vi "ROSPublisher.vi"(2 "Response":T1, 3 "ROS":T2={"topic port"=1236, "Node"="/labview", "topic"="/robot/head/command_head_nod", "type"="std_msgs/Bool", "node port"=7000, "error "={"status"=FALSE, "code"=0, "source"=""}, "Direction"=enum."Publisher", "Update (ms)"=1, "FIFO size"=1}) -> ()   [LabVIEW 2012]
doc: "Opens new ports for publishers, updates publishers with master, and closes publishers"
uses:
  <userlib>/ROS for LabVIEW Software/ROS/Code/SubVIs/_ROSControl.ctl
  <userlib>/ROS for LabVIEW Software/ROS/Code/SubVIs/_ROSDirection.ctl
  <userlib>/ROS for LabVIEW Software/ROS/Code/_ROSDefinition.vi
panel:
  out "ports":i32[](array[numeric])
  out "Queue log":string
  out "Watchdog":i32
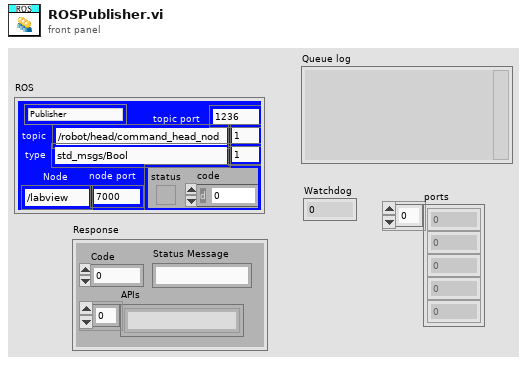
[diagram p1: front panel]
types:
  T1 = cluster{"Code":i32, "Status Message":string, "APIs":string[]}
  T2 = typedef "_ROSControl.ctl" = cluster{"topic port":u16, "Node":string, "topic":string, "type":string, "node port":u16, "error ":errorcluster, "Direction":T3, "Update (ms)":u16, "FIFO size":u16}
  T3 = typedef "_ROSDirection.ctl" = enum16{"Node", "Publisher", "Subscriber", "ServiceClient", "ServiceProvider"}
  T4 = enum16{"Reset Log", "Add Client", "Remove Client", "Add Task"}
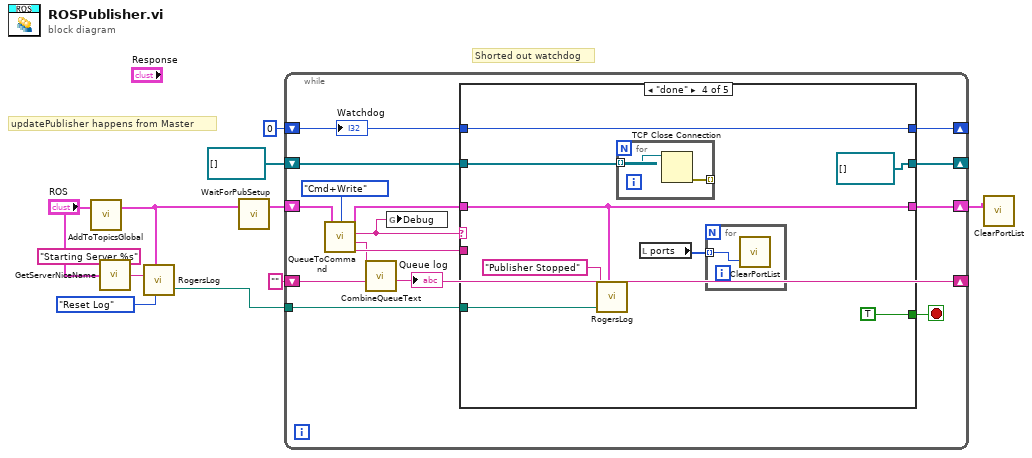
[diagram p0: block diagram]
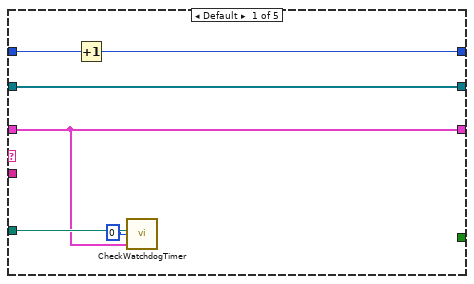
[diagram p2: hidden frame]
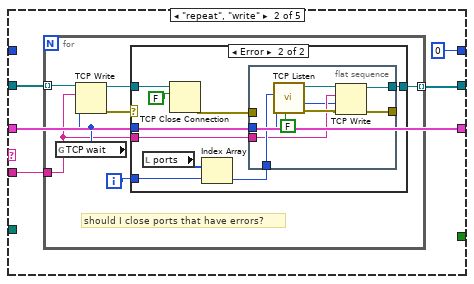
[diagram p3: hidden frame]
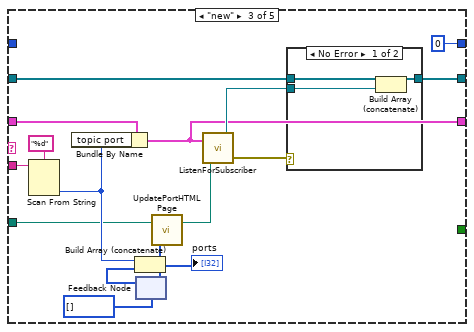
[diagram p5: hidden frame]
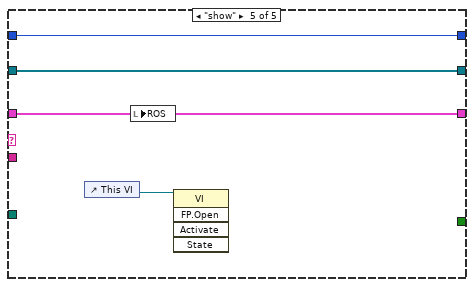
[diagram p7: hidden frame]
diagram:
  # "Shorted out watchdog"
  # "updatePublisher happens from Master"
  n1 = call <userlib>:"AddToTopicsGlobal.vi"("ROS in"="ROS") -> ("ROS out"=w1:T2)  [unwired: 2 in]
  n2 = call <userlib>:"GetServerNiceName.vi"("ROS"="ROS", "Text to add"="Starting Server %s") -> ("String"=w10:string)
  n3 = call <userlib>:"RogersLog.vi"("Text to add"=w10, "ROS"=w1, "Task"=T4."Reset Log") -> ("LogPath out"=w7:path)  [unwired: 2 in, 1 out]
  n4 = call <userlib>:"WaitForPubSetup.vi"("ROS in"=w1) -> ("ROS out"=w5:T2)  [unwired: 2 in]
  n5 = while {
    tunnel: w7 -> [w23]
    shift-right: [w21] -> _
    shift-left: 0 ("timeout ms (wait forever: -1)") -> [w22]
    shift-right: [w20] -> _
    shift-left: refnum<k5>[] [] -> [w26]
    shift-right: [w17] -> _
    shift-left: "" ("New List") -> [w19]
    shift-right: [w14] -> w2
    shift-left: w5 -> [w16]
    stop <- w24 stop-if-true
    n6 = call <userlib>:"QueueToCommand.vi"("ROS"=w16, "Check"=enum16{"Cmd+Write", "FIFO", "CMD", "CMD /wait"}."Cmd+Write") -> ("ROS out"=w15:T2, "Command"=w12:string, "Queue log"=w18:string, "data"=w25:string)  [unwired: 1 in]
    n7 = call <userlib>:"CombineQueueText.vi"("Old List"=w19, "Queue In"=w18) -> ("New List"=w17:string)  [unwired: 1 in]
    "Queue log" <- w17
    n8 = global write "_ROSDefinition.vi" "Debug"(w12) -> ()
    n9 = case shown="\"done\"" w12 {
      tunnel: w26 -> [w31 w36 w74 w84 w94]
      tunnel: w25 -> [_ w33 w76 _ _]
      tunnel: [_ _ _ TRUE _] -> w24
      tunnel: w23 -> [w29 _ w65 w88 _]
      tunnel: w22 -> [w32 _ _ w86 w95]
      tunnel: [w30 0 ("timeout ms (wait forever: -1)") 0 ("timeout ms (wait forever: -1)") w86 w95] -> w21
      tunnel: w15 -> [w27 w34 w67 w82 w93]
      tunnel: [w31 w35 w72 refnum<k5>[] [] w94] -> w20
      tunnel: [w27 w34 w63 w82 w93] -> w14
      frame Default {
        n10 = Increment(x=w32) -> (x+1=w30:i32)
        n11 = call <userlib>:"CheckWatchdogTimer.vi"("ROS"=w27, "itteration"=0, "LogPath in"=w29) -> ()  [unwired: 3 in]
      }
      frame "repeat", "write" {
        n12 = for {
          tunnel: w36 -> [w44] mode=indexing
          tunnel: w33 -> [w38]
          tunnel: [w41] -> w35 mode=indexing
          i -> [w40]
          # "should I close ports that have errors?"
          n13 = global read "_ROSDefinition.vi" "TCP wait"() -> (w39:i32)
          n14 = TCP Write(connection ID=w44, data in=w38, 9:w39) -> (connection ID out=w42:refnum<k5>, error out=w43:errorcluster)  [unwired: 1 in, 1 out]
          n15 = case shown="Error" w43 {
            tunnel: w42 -> [w45 w54]
            tunnel: [w45 w52] -> w41
            tunnel: w40 -> [_ w50]
            tunnel: w39 -> [_ w47]
            tunnel: w38 -> [_ w46]
            frame No Error {
            }
            frame Error {
              n16 = local read "ports"() -> (w51:i32[])
              n17 = TCP Close Connection(connection ID=w54, abort (F)=FALSE) -> (error out=w48:errorcluster)  [unwired: 1 in, 1 out]
              n18 = Index Array(array=w51, index=w50) -> (element=w49:i32)
              n19 = flat-sequence {
                tunnel: [w58] -> w52
                tunnel: w49 -> [w62]
                tunnel: w47 -> [w55]
                tunnel: w48 -> [_]
                tunnel: [w60] -> _
                tunnel: w46 -> [w57]
                frame #0 {
                  n20 = call <vilib>:"TCP Listen.vi"("resolve remote address (T)"=FALSE, "timeout ms (wait forever: -1)"=w55, "port"=w62) -> ("error out"=w61:errorcluster, "connection ID"=w59:refnum<k5>)  [unwired: 4 in, 3 out]
                  n21 = TCP Write(connection ID=w59, data in=w57, error in (no error)=w61, 9:w55) -> (connection ID out=w58:refnum<k5>, error out=w60:errorcluster)  [unwired: 1 out]
                }
              }
            }
          }
        }
      }
      frame "new" {
        n22 = Scan From String(format string="%d", input string=w76) -> (output 1=w70:i32)  [unwired: 3 in, 3 out]
        n23 = Bundle By Name(cluster=w67, "topic port"=w70) -> (w63:T2)
        n24 = feedback #1(i32[] []) -> (w69:i32[])
        n25 = Build Array (concatenate)(w70, w69) -> (w64:i32[])
        "ports" <- w64
        n26 = feedback-in #1(w64) -> ()
        n27 = call <userlib>:"UpdatePortHTMLPage.vi"("Array"=w64, "LogPath in"=w65) -> ("LogPath out"=w66:path)  [unwired: 1 in]
        n28 = call <userlib>:"ListenForSubscriber.vi"("LogPath in"=w66, "ROS"=w63) -> ("heard?"=w71:errorcluster, "server"=w73:refnum<k5>)
        n29 = case shown="No Error" w71 {
          tunnel: w74 -> [w80 w81]
          tunnel: w73 -> [w79 _]
          tunnel: [w78 w81] -> w72
          frame No Error {
            n30 = Build Array (concatenate)(w80, w79) -> (w78:refnum<k5>[])
          }
          frame Error {
          }
        }
      }
      frame "done" {
        n31 = call <userlib>:"RogersLog.vi"("Text to add"="Publisher Stopped", "ROS"=w82, "LogPath in"=w88) -> ()  [unwired: 2 in, 2 out]
        n32 = for {
          tunnel: w84 -> [w91] mode=indexing
          tunnel: [w90] -> _ mode=indexing
          n33 = TCP Close Connection(connection ID=w91) -> (error out=w90:errorcluster)  [unwired: 2 in, 1 out]
        }
        n34 = local read "ports"() -> (w85:i32[])
        n35 = for {
          tunnel: w85 -> [w92] mode=indexing
          n36 = call <userlib>:"ClearPortList.vi"("topic port"=w92) -> ()  [unwired: 2 in]
        }
      }
      frame "show" {
        n37 = control-ref of="This VI"() -> (w96:refnum<vi>)
        n38 = local write "ROS"(w93) -> ()
        n39 = invoke class="VI" method="FP.Open"(reference=w96) -> ()  [unwired: 4 in, 5 out]
      }
    }
    "Watchdog" <- w22
  }
  n40 = call <userlib>:"ClearPortList.vi"("ROS"=w2) -> ()  [unwired: 2 in]
